vi "RichToFlatw4lvgrpc_ToClient.vi"(5 "OutputClusterType":T1, 11 "InputCluster":T11) -> (3 "OutputCluster":T1)   [LabVIEW 2019, in "Generated_server.lvlib"]
uses:
  Generated_server.lvlib
  w4lvgrpc_ToClient_payload/w4lvgrpc_ToClient_payload.lvclass
  w4lvgrpc_Msg_ToClient_9_Flat.ctl
  w4lvgrpc_Msg_ToClient_8_Flat.ctl
  w4lvgrpc_Msg_ToClient_7_Flat.ctl
  w4lvgrpc_Msg_ToClient_6_Flat.ctl
  w4lvgrpc_Msg_ToClient_5_Flat.ctl
  w4lvgrpc_Msg_ToClient_4_Flat.ctl
  w4lvgrpc_Msg_ToClient_3_Flat.ctl
  w4lvgrpc_Msg_ToClient_2_Flat.ctl
  w4lvgrpc_Msg_ToClient_1_Flat.ctl
  w4lvgrpc_ToClient_Flat.ctl
  w4lvgrpc_ToClient.ctl
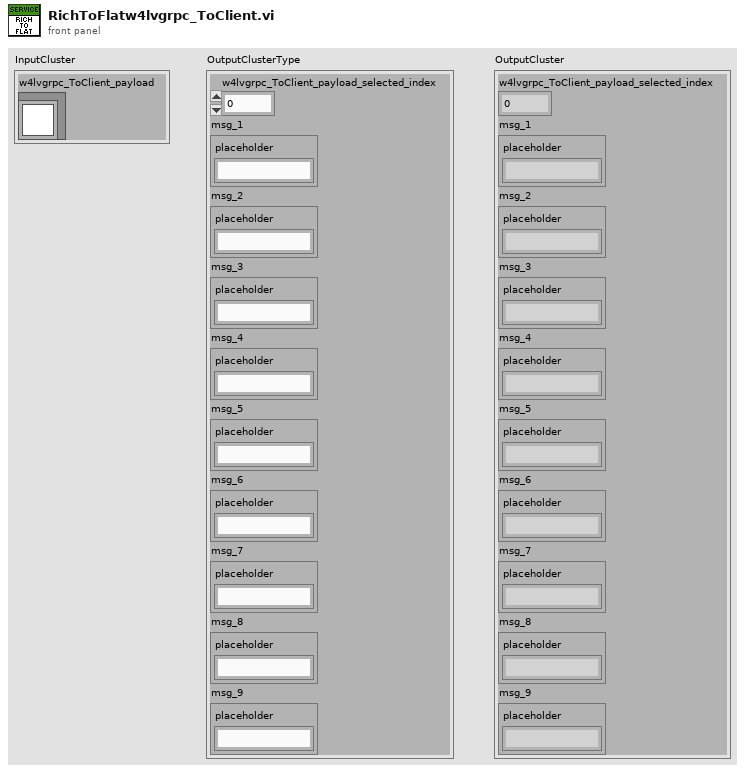
[diagram p1: front panel]
types:
  T1 = typedef "Generated_server.lvlib/w4lvgrpc_ToClient_Flat.ctl" = cluster{"w4lvgrpc_ToClient_payload_selected_index":i32, "msg_1":T2, "msg_2":T3, "msg_3":T4, "msg_4":T5, "msg_5":T6, "msg_6":T7, "msg_7":T8, "msg_8":T9, "msg_9":T10}
  T2 = typedef "Generated_server.lvlib/w4lvgrpc_Msg_ToClient_1_Flat.ctl" = cluster{"placeholder":string}
  T3 = typedef "Generated_server.lvlib/w4lvgrpc_Msg_ToClient_2_Flat.ctl" = cluster{"placeholder":string}
  T4 = typedef "Generated_server.lvlib/w4lvgrpc_Msg_ToClient_3_Flat.ctl" = cluster{"placeholder":string}
  T5 = typedef "Generated_server.lvlib/w4lvgrpc_Msg_ToClient_4_Flat.ctl" = cluster{"placeholder":string}
  T6 = typedef "Generated_server.lvlib/w4lvgrpc_Msg_ToClient_5_Flat.ctl" = cluster{"placeholder":string}
  T7 = typedef "Generated_server.lvlib/w4lvgrpc_Msg_ToClient_6_Flat.ctl" = cluster{"placeholder":string}
  T8 = typedef "Generated_server.lvlib/w4lvgrpc_Msg_ToClient_7_Flat.ctl" = cluster{"placeholder":string}
  T9 = typedef "Generated_server.lvlib/w4lvgrpc_Msg_ToClient_8_Flat.ctl" = cluster{"placeholder":string}
  T10 = typedef "Generated_server.lvlib/w4lvgrpc_Msg_ToClient_9_Flat.ctl" = cluster{"placeholder":string}
  T11 = typedef "Generated_server.lvlib/w4lvgrpc_ToClient.ctl" = cluster{"w4lvgrpc_ToClient_payload":refnum<class "w4lvgrpc_ToClient_payload.lvclass">}
  T12 = typedef "Generated_server.lvlib/w4lvgrpc_Msg_ToClient_1.ctl" = cluster{"placeholder":string}
  T13 = typedef "Generated_server.lvlib/w4lvgrpc_Msg_ToClient_2.ctl" = cluster{"placeholder":string}
  T14 = typedef "Generated_server.lvlib/w4lvgrpc_Msg_ToClient_3.ctl" = cluster{"placeholder":string}
  T15 = typedef "Generated_server.lvlib/w4lvgrpc_Msg_ToClient_4.ctl" = cluster{"placeholder":string}
  T16 = typedef "Generated_server.lvlib/w4lvgrpc_Msg_ToClient_5.ctl" = cluster{"placeholder":string}
  T17 = typedef "Generated_server.lvlib/w4lvgrpc_Msg_ToClient_6.ctl" = cluster{"placeholder":string}
  T18 = typedef "Generated_server.lvlib/w4lvgrpc_Msg_ToClient_7.ctl" = cluster{"placeholder":string}
  T19 = typedef "Generated_server.lvlib/w4lvgrpc_Msg_ToClient_8.ctl" = cluster{"placeholder":string}
  T20 = typedef "Generated_server.lvlib/w4lvgrpc_Msg_ToClient_9.ctl" = cluster{"placeholder":string}
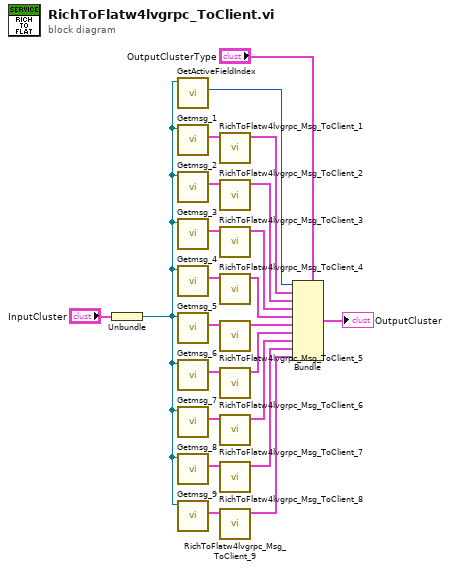
[diagram p0: block diagram]
diagram:
  n1 = Unbundle "Unbundle"("InputCluster") -> ("w4lvgrpc_ToClient_payload"=w20:refnum<class "w4lvgrpc_ToClient_payload.lvclass">)
  n2 = call "GetActiveFieldIndex.vi"("OneOfTemplate in"=w20) -> ("Active Field Index"=w19:i32)  [unwired: 8 in, 2 out]
  n3 = call "Getmsg_1.vi"("OneOfTemplate in"=w20) -> ("Get_Val"=w18:T12)  [unwired: 8 in, 2 out]
  n4 = call "Getmsg_2.vi"("OneOfTemplate in"=w20) -> ("Get_Val"=w16:T13)  [unwired: 8 in, 2 out]
  n5 = call "Getmsg_3.vi"("OneOfTemplate in"=w20) -> ("Get_Val"=w14:T14)  [unwired: 8 in, 2 out]
  n6 = call "Getmsg_4.vi"("OneOfTemplate in"=w20) -> ("Get_Val"=w12:T15)  [unwired: 8 in, 2 out]
  n7 = call "Getmsg_5.vi"("OneOfTemplate in"=w20) -> ("Get_Val"=w10:T16)  [unwired: 8 in, 2 out]
  n8 = call "Getmsg_6.vi"("OneOfTemplate in"=w20) -> ("Get_Val"=w8:T17)  [unwired: 8 in, 2 out]
  n9 = call "Getmsg_7.vi"("OneOfTemplate in"=w20) -> ("Get_Val"=w6:T18)  [unwired: 8 in, 2 out]
  n10 = call "Getmsg_8.vi"("OneOfTemplate in"=w20) -> ("Get_Val"=w4:T19)  [unwired: 8 in, 2 out]
  n11 = call "Getmsg_9.vi"("OneOfTemplate in"=w20) -> ("Get_Val"=w2:T20)  [unwired: 8 in, 2 out]
  n12 = call "RichToFlatw4lvgrpc_Msg_ToClient_1.vi"("InputCluster"=w18) -> ("OutputCluster"=w17:T2)  [unwired: 10 in]
  n13 = call "RichToFlatw4lvgrpc_Msg_ToClient_2.vi"("InputCluster"=w16) -> ("OutputCluster"=w15:T3)  [unwired: 10 in]
  n14 = call "RichToFlatw4lvgrpc_Msg_ToClient_3.vi"("InputCluster"=w14) -> ("OutputCluster"=w13:T4)  [unwired: 10 in]
  n15 = call "RichToFlatw4lvgrpc_Msg_ToClient_4.vi"("InputCluster"=w12) -> ("OutputCluster"=w11:T5)  [unwired: 10 in]
  n16 = call "RichToFlatw4lvgrpc_Msg_ToClient_5.vi"("InputCluster"=w10) -> ("OutputCluster"=w9:T6)  [unwired: 10 in]
  n17 = call "RichToFlatw4lvgrpc_Msg_ToClient_6.vi"("InputCluster"=w8) -> ("OutputCluster"=w7:T7)  [unwired: 10 in]
  n18 = call "RichToFlatw4lvgrpc_Msg_ToClient_7.vi"("InputCluster"=w6) -> ("OutputCluster"=w5:T8)  [unwired: 10 in]
  n19 = call "RichToFlatw4lvgrpc_Msg_ToClient_8.vi"("InputCluster"=w4) -> ("OutputCluster"=w3:T9)  [unwired: 10 in]
  n20 = call "RichToFlatw4lvgrpc_Msg_ToClient_9.vi"("InputCluster"=w2) -> ("OutputCluster"=w1:T10)  [unwired: 10 in]
  n21 = Bundle "Bundle"(cluster="OutputClusterType", "w4lvgrpc_ToClient_payload_selected_index"=w19, "msg_1"=w17, "msg_2"=w15, "msg_3"=w13, "msg_4"=w11, "msg_5"=w9, "msg_6"=w7, "msg_7"=w5, "msg_8"=w3, "msg_9"=w1) -> (→"OutputCluster":T1)
